vi "String to Boolean.vi"(11 "String":string="RLR") -> (0 "Boolean Array":bool[](array[boolean]))   [LabVIEW 2017]
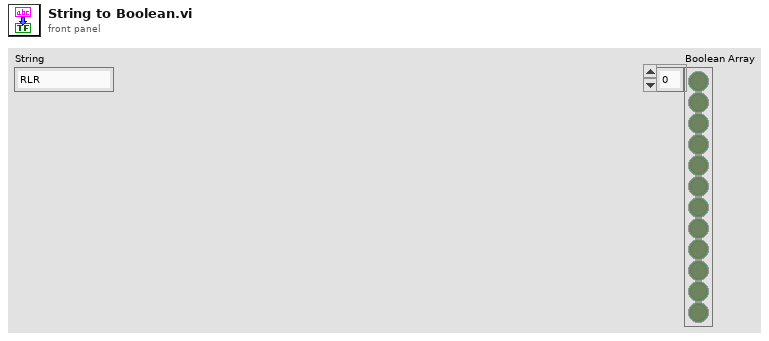
[diagram p1: front panel]
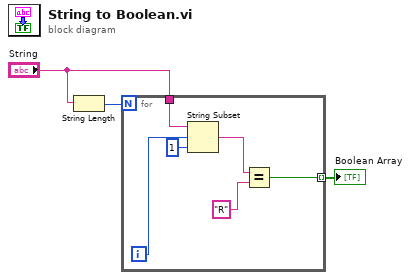
[diagram p0: block diagram]
diagram:
  n1 = String Length(string="String") -> (length=w2:i32)
  n2 = for {
    N: w2 -> [_]
    tunnel: "String" -> [w9]
    tunnel: [w4] -> w3 mode=indexing
    i -> [w8]
    n3 = String Subset(string=w9, offset (0)=w8, length (rest)=1 ("length (rest)")) -> (substring=w6:string)
    n4 = Equal?(x=w6, y="R") -> (x = y?=w4:bool)
  }
  "Boolean Array" <- w3
